vi "interfaceLoop systemRecord.vi"(7 "Version :":refnum<vi>, 8 "error in (no error)":errorcluster, 9 "connectStateRefnum":refnum<data-value>, 11 "Stop":refnum<vi>) -> (0 "error out":errorcluster)   [LabVIEW 2018]
uses:
  <vilib>/Platform/TimedLoop/XDataNode/timing_clust.ctl
  <vilib>/Platform/TimedLoop/XDataNode/nitl_modes.ctl
  <vilib>/Platform/TimedLoop/XDataNode/wakeup.ctl
  <vilib>/Platform/TimedLoop/XDataNode/XDataNode.xnode
  <vilib>/Platform/TimedLoop/XDataNode/XDNodeRunTimeDep.lvlib
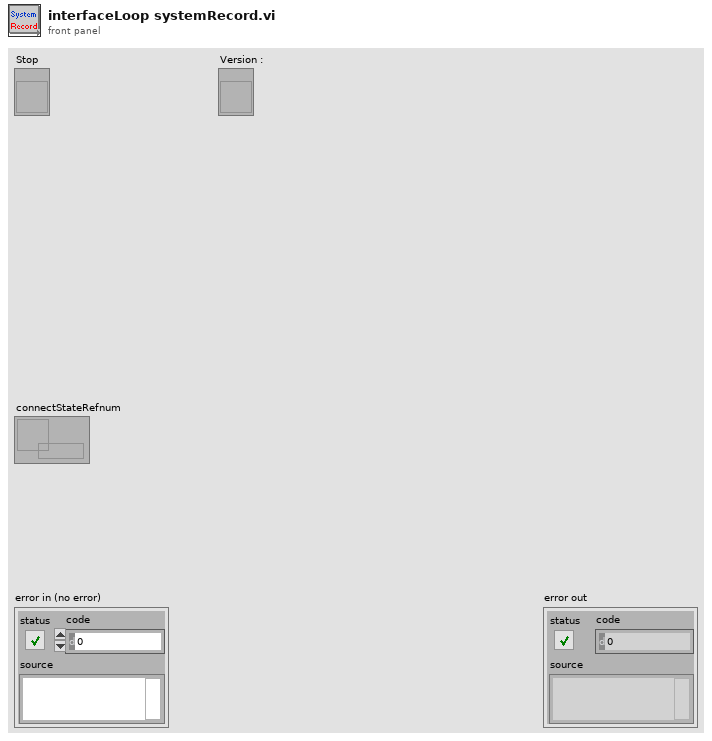
[diagram p1: front panel]
types:
  T1 = typedef "XDNodeRunTimeDep.lvlib/timing_clust.ctl" = cluster{"Expected End [f-1]":u64, "Actual End [f-1]":u64, "Finished Late? [f-1]":bool, "Expected End [i-1]":u64, "Actual End [i-1]":u64, "Finished Late? [i-1]":bool, "Expected Start [i]":u64, "Actual Start [i]":u64, "Expected Start [f]":u64, "Actual Start [f]":u64, "Source Name":string, "Structure Name":string, "Period":i64, "Deadline":i64, "Offset":i64, "Start":i64, "Priority":i32, "Timeout":i32, "Mode":T2, "Wakeup Reason":T3, "Error":errorcluster, "Source Type":string, "Secondary Source Type":string, "Global End Time":u64, "Global Start Time":u64, "Frame Duration":u64, "Iteration Duration":u64, "Assigned CPU":i32, "I/O Scan Engine Mode":u32}
  T2 = typedef "XDNodeRunTimeDep.lvlib/nitl_modes.ctl" = enum32{"No Change", "Process missed periods, maintain original phase", "Discard missed periods, maintain original phase", "Process missed periods, ignore original phase", "Discard missed periods, ignore original phase"}
  T3 = typedef "XDNodeRunTimeDep.lvlib/wakeup.ctl" = enum32{"Normal", "Aborted", "Asynchronous wakeup", "Timing source error", "Timed loop error", "Timeout"}
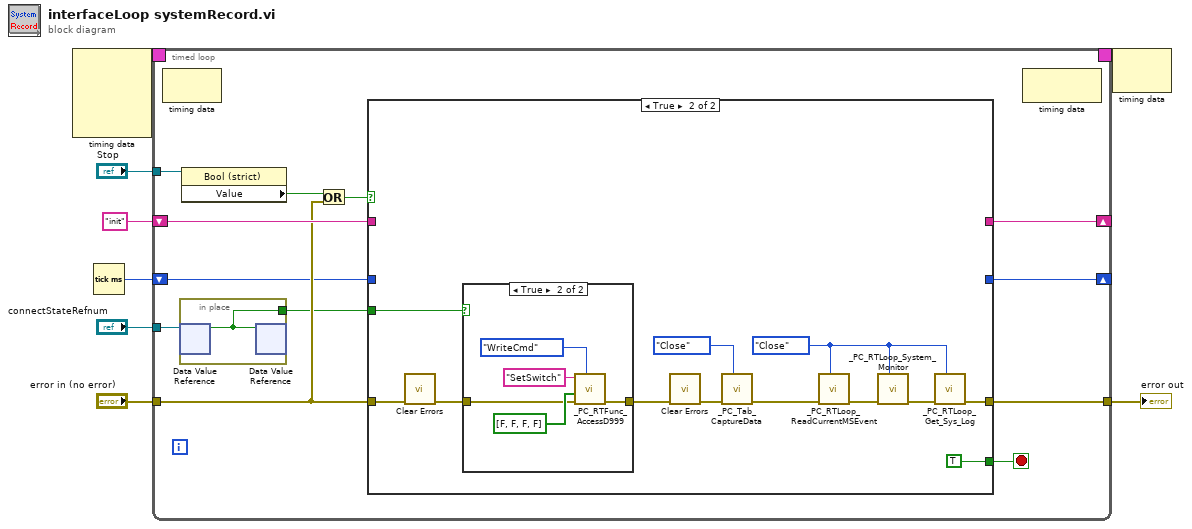
[diagram p0: block diagram]
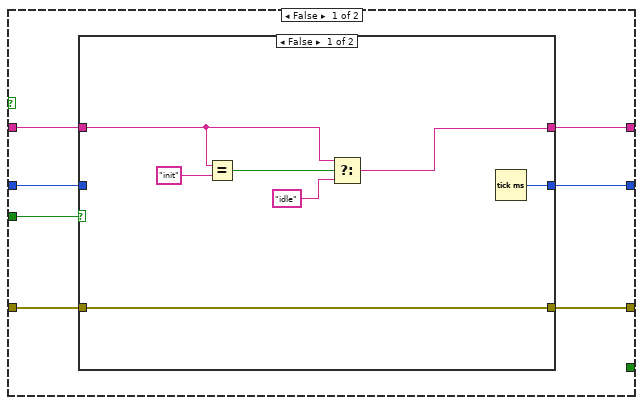
[diagram p2: hidden frame]
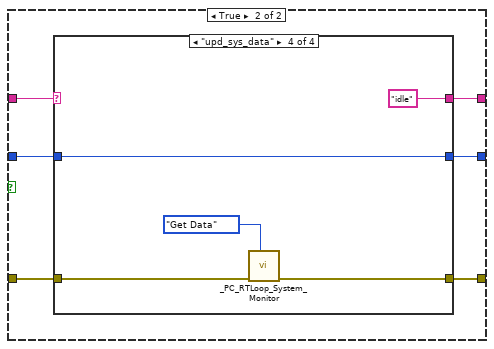
[diagram p3: hidden frame]
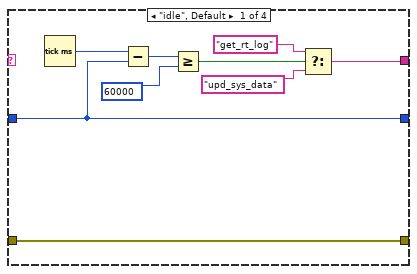
[diagram p4: hidden frame]
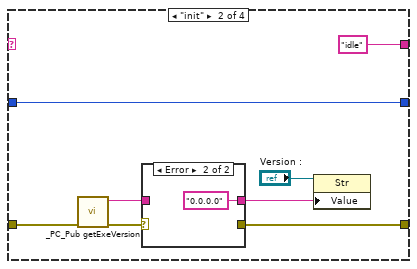
[diagram p5: hidden frame]
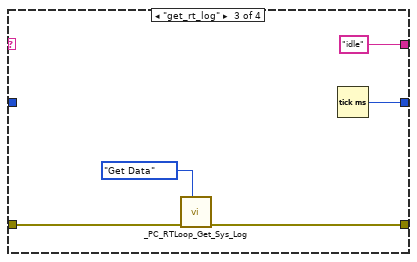
[diagram p7: hidden frame]
diagram:
  n1 = node-c288() -> (w2:T1)  [unwired: 4 in]
  n2 = Tick Count (ms)() -> (millisecond timer value=w4:u32)
  n3 = timed-loop {
    tunnel: "Stop" -> [w20]
    shift-right: [w13] -> _
    shift-left: "init" ("t") -> [w17]
    tunnel: "connectStateRefnum" -> [w15]
    tunnel: "error in (no error)" -> [w16]
    shift-right: [w11] -> _
    shift-left: w4 -> [w12]
    tunnel: [w9] -> w3
    timing: w2 -> [_]
    timing-out: [_] -> w1
    stop <- w10 stop-if-true
    n4 = node-c288() -> ()  [unwired: 1 in, 1 out]
    n5 = in-place {
      in-place-border: [w23] -> w14
      n6 = in-place-dvr #1(w15) -> (w23:bool)  [unwired: 1 out]
      n7 = in-place-dvr #1(w23) -> ()  [unwired: 2 out]
    }
    n8 = property class="Bool (strict)"(reference=w20) -> ("Value"=w19:bool)  [unwired: 1 in, 2 out]
    n9 = Or(x=w19, y=w16) -> (x .or. y?=w18:bool)
    n10 = case shown="True" w18 {
      tunnel: w17 -> [w30 _]
      tunnel: w16 -> [w28 w85]
      tunnel: [w27 w76] -> w9
      tunnel: w14 -> [w29 w75]
      tunnel: [w26 _] -> w13
      tunnel: w12 -> [w25 _]
      tunnel: [w24 _] -> w11
      tunnel: [_ TRUE] -> w10
      frame False {
        n11 = case shown="False" w29 {
          tunnel: w30 -> [w33 w43]
          tunnel: w28 -> [w37 w42]
          tunnel: [w37 w41] -> w27
          tunnel: [w31 w40] -> w26
          tunnel: w25 -> [_ w39]
          tunnel: [w36 w38] -> w24
          frame False {
            n12 = Equal?(x=w33, y="init") -> (x = y?=w34:bool)
            n13 = Select(t=w33, s=w34, f="idle") -> (s? t:f=w31:string)
            n14 = Tick Count (ms)() -> (millisecond timer value=w36:u32)
          }
          frame True {
            n15 = case shown="\"upd_sys_data\"" w43 {
              tunnel: w42 -> [w44 w56 w67 w72]
              tunnel: [w44 w55 w66 w71] -> w41
              tunnel: [w50 "idle" ("t") "idle" ("t") "idle" ("t")] -> w40
              tunnel: w39 -> [w45 w53 _ w69]
              tunnel: [w45 w53 w64 w69] -> w38
              frame "idle", Default {
                n16 = Tick Count (ms)() -> (millisecond timer value=w49:u32)
                n17 = Subtract(x=w49, y=w45) -> (x-y=w48:u32)
                n18 = Greater Or Equal?(x=w48, y=u32 60000) -> (x >= y?=w46:bool)
                n19 = Select(t="get_rt_log" ("element"), s=w46, f="upd_sys_data" ("element")) -> (s? t:f=w50:string)
              }
              frame "init" {
                n20 = call "_PC_Pub getExeVersion.vi"("error in (no error)"=w56) -> ("error out"=w60:errorcluster, "version serial number"=w59:string)  [unwired: 8 in, 1 out]
                n21 = case shown="Error" w60 {
                  selector: w60 -> [w61 _]
                  tunnel: [w62 "0.0.0.0" ("version serial number")] -> w57
                  tunnel: w59 -> [w62 _]
                  tunnel: [w61 _] -> w55
                  frame No Error {
                  }
                  frame Error {
                  }
                }
                n22 = property class="Str"(reference="Version :", "Value"=w57) -> ()  [unwired: 1 in, 2 out]
              }
              frame "get_rt_log" {
                n23 = call "_PC_RTLoop_Get_Sys_Log.vi"("Function"=enum16{"Init", "Get Data", "Close"}."Get Data", "error in (no error)"=w67) -> ("error out"=w66:errorcluster)  [unwired: 9 in]
                n24 = Tick Count (ms)() -> (millisecond timer value=w64:u32)
              }
              frame "upd_sys_data" {
                n25 = call "_PC_RTLoop_System_Monitor.vi"("Function"=enum16{"Init", "Get Data", "Close"}."Get Data", "error in (no error)"=w72) -> ("error out"=w71:errorcluster)  [unwired: 9 in]
              }
            }
          }
        }
      }
      frame True {
        w77 = enum16{"Init", "Get Data", "Close"}."Close" ("Function")
        n26 = call <vilib>:"Clear Errors.vi"("error in (no error)"=w85) -> ("error out"=w84:errorcluster)  [unwired: 5 in, 1 out]
        n27 = case shown="True" w75 {
          tunnel: w84 -> [w86 w89]
          tunnel: [w86 w88] -> w82
          frame False {
          }
          frame True {
            n28 = call "_PC_RTFunc_AccessD999.vi"("Function"=enum16{"WriteCmd", "ReadParam", "ReadResponse"}."WriteCmd", "error in (no error)"=w89, "Variant"=bool[] [FALSE, FALSE, FALSE, FALSE], "Cmd"="SetSwitch") -> ("error out"=w88:errorcluster)  [unwired: 6 in, 1 out]
          }
        }
        n29 = call <vilib>:"Clear Errors.vi"("error in (no error)"=w82) -> ("error out"=w81:errorcluster)  [unwired: 5 in, 1 out]
        n30 = call "_PC_Tab_CaptureData.vi"("Function"=enum16{"Init", "Get Data", "Update", "Close"}."Close", "error in (no error)"=w81) -> ("error out"=w80:errorcluster)  [unwired: 9 in]
        n31 = call "_PC_RTLoop_ReadCurrentMSEvent.vi"("Function"=w77, "error in (no error)"=w80) -> ("error out"=w79:errorcluster)  [unwired: 9 in]
        n32 = call "_PC_RTLoop_System_Monitor.vi"("Function"=w77, "error in (no error)"=w79) -> ("error out"=w78:errorcluster)  [unwired: 9 in]
        n33 = call "_PC_RTLoop_Get_Sys_Log.vi"("Function"=w77, "error in (no error)"=w78) -> ("error out"=w76:errorcluster)  [unwired: 9 in]
      }
    }
    n34 = node-c288() -> ()  [unwired: 1 in, 1 out]
  }
  "error out" <- w3
  n35 = node-c288(w1) -> ()  [unwired: 1 out]
